vi "GUI Final.vi"() -> ()   [LabVIEW 2014]
uses:
  <vilib>/Instr/_visa.llb/VISA Configure Serial Port (Instr).vi
panel:
  in  "Temperature Threshold":string
  out "read buffer":string
  out "pass ACK":bool
  out "Threshold sent":bool
  out "no of trials read":bool
  out "PC on Ack":bool
  out "Reset#":i32
  in  "Reset":bool
  out "return count read":u32
  in  "VISA resource name":refnum<visa-resource-name>
  out "Iteration":i32
  out "password is wrong":bool
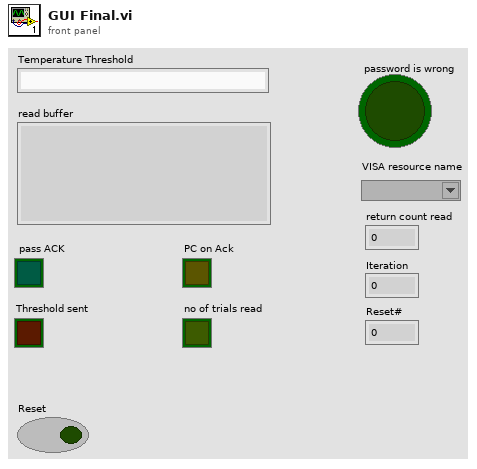
[diagram p1: front panel]
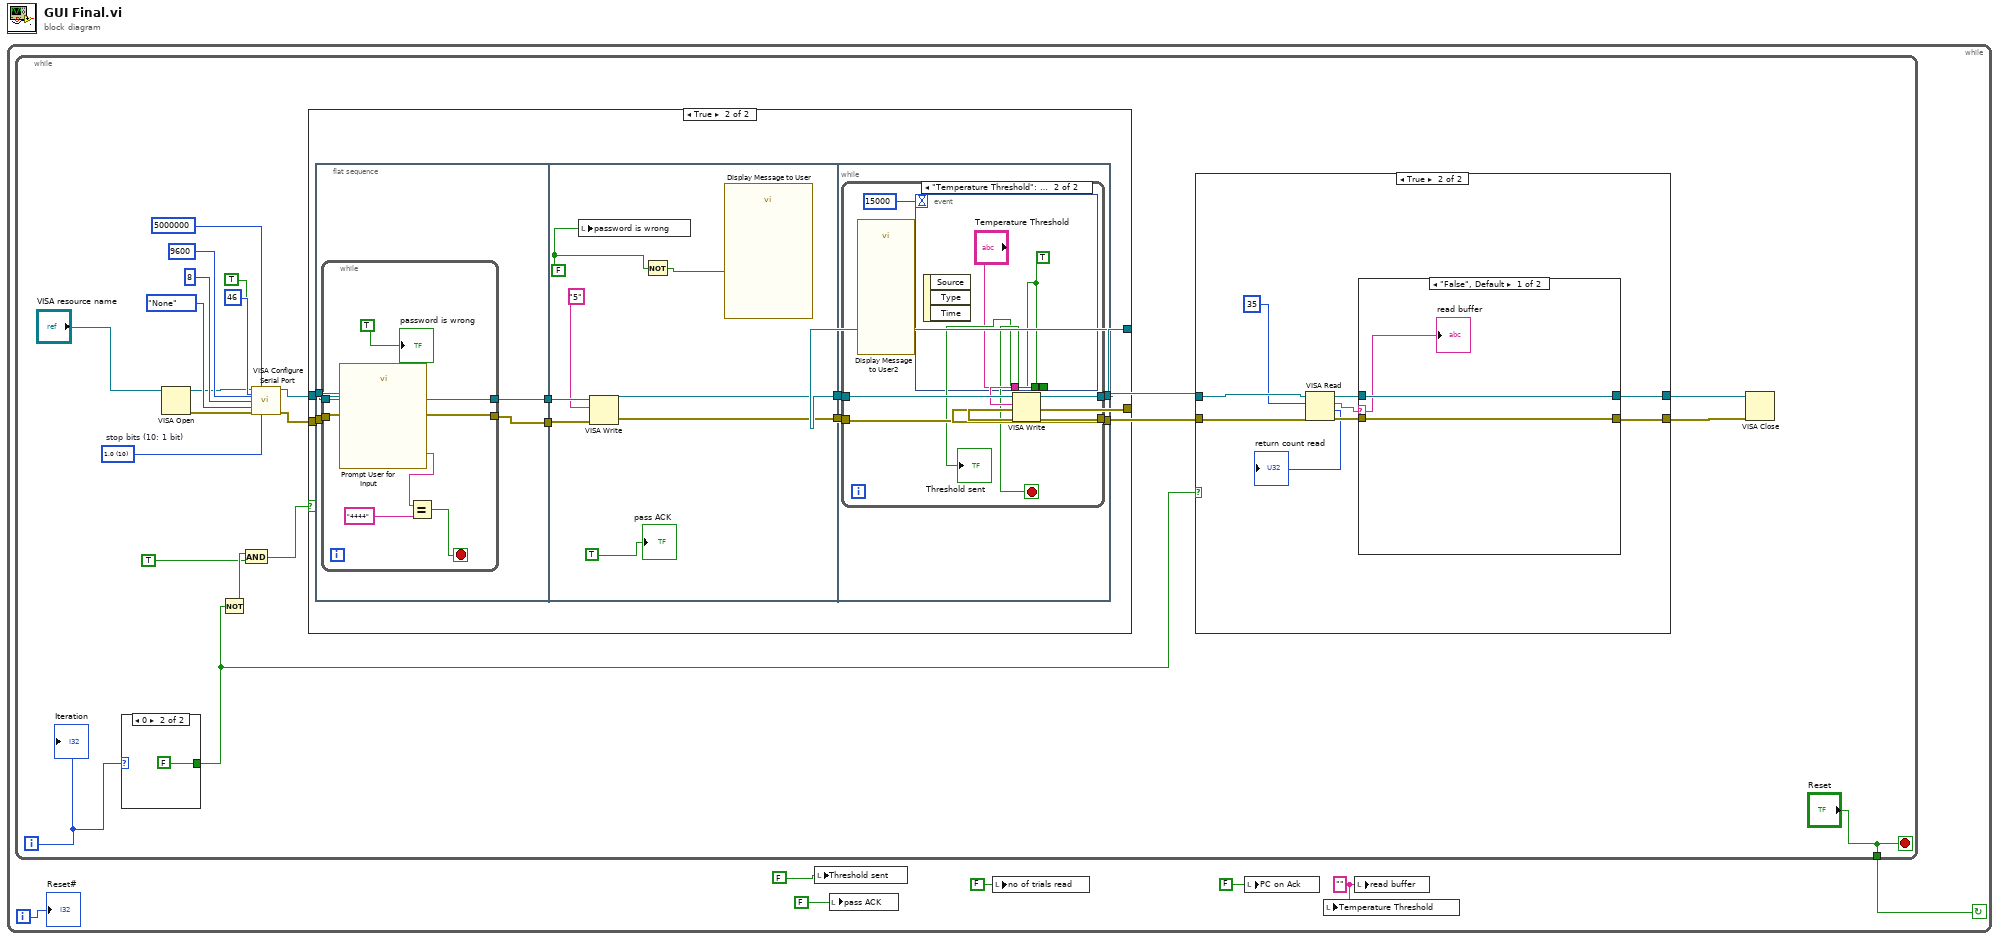
[diagram p0: block diagram]
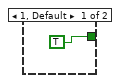
[diagram p2: hidden frame]
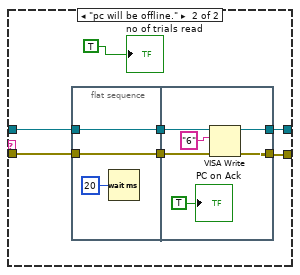
[diagram p4: hidden frame]
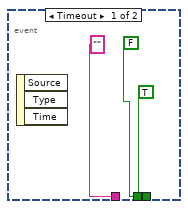
[diagram p6: hidden frame]
diagram:
  n1 = while {
    i -> [w7]
    stop <- w6 continue-if-true
    w1 = "" ("read buffer")
    n2 = while {
      tunnel: ["Reset"] -> w6
      i -> [w15]
      stop <- "Reset" stop-if-true
      w26 = u16 10 items=["1.0"=10, "1.5"=15, "2.0"=20]  # stop bits (10: 1 bit)
      n3 = case shown="0" w15 {
        tunnel: [TRUE FALSE] -> w14
        frame 1, Default {
        }
        frame 0 {
        }
      }
      n4 = VISA Open(VISA resource name="VISA resource name") -> (VISA resource name=w10:refnum<visa-resource-name>, error out=w9:errorcluster)  [unwired: 4 in]
      n5 = Not(x=w14) -> (.not. x?=w23:bool)
      n6 = And(x=w23, y=TRUE) -> (x .and. y?=w20:bool)
      n7 = call-poly "VISA Configure Serial Port"("VISA resource name"=w10, "timeout (10sec)"=u32 5000000, "termination char\n(0xA = '\\n' = LF)"=u8 46 ("termination char\n(0xA = '\\n' = LF)"), "Enable Termination\nChar (T)"=TRUE ("Enable Termination\nChar (T)"), "baud rate (9600)"=u32 9600, "data bits (8)"=u16 8, "parity (0:none)"=enum16{"None", "Odd", "Even", "Mark", "Space"}."None", "error in (no error)"=w9, "stop bits (10: 1 bit)"=w26) -> ("VISA resource name out"=w22:refnum<visa-resource-name>, "error out"=w21:errorcluster)  [unwired: 5 in]
      n8 = case shown="True" w20 {
        tunnel: w21 -> [w63 w71]
        tunnel: [w62 w69] -> w19
        tunnel: [w63 w68] -> w17
        tunnel: w22 -> [w62 w70]
        frame False {
        }
        frame True {
          n9 = flat-sequence {
            tunnel: w71 -> [w75]
            tunnel: w70 -> [w74]
            tunnel: [w73] -> w65
            tunnel: [w72] -> w64
            tunnel: w65 -> [w89]
            tunnel: w64 -> [w88]
            tunnel: [w87] -> w67
            tunnel: [w86] -> w66
            tunnel: [w92] -> w69
            tunnel: [w91] -> w68
            tunnel: w67 -> [w93]
            tunnel: w66 -> [w90]
            frame #0 {
              n10 = while {
                tunnel: w75 -> [w80]
                tunnel: w74 -> [w79]
                tunnel: [w80] -> w73
                tunnel: [w79] -> w72
                stop <- w81 stop-if-true
                n11 = call "Prompt User for Input"() -> ("password"=w76:string)  [unwired: 17 in, 2 out]
                n12 = Equal?(x=w76, y="4444") -> (x = y?=w81:bool)
                "password is wrong" <- TRUE
              }
            }
            frame #1 {
              w83 = FALSE
              n13 = local write "password is wrong"(w83) -> ()
              n14 = VISA Write(VISA resource name=w88, write buffer="5", error in (no error)=w89) -> (VISA resource name out=w87:refnum<visa-resource-name>, error out=w86:errorcluster)  [unwired: 1 out]
              n15 = Not(x=w83) -> (.not. x?=w82:bool)
              n16 = call "Display Message to User"("Enable"=w82) -> ()  [unwired: 9 in, 2 out]
              "pass ACK" <- TRUE ("Pass Ack")
            }
            frame #2 {
              n17 = while {
                tunnel: w93 -> [w101]
                tunnel: [w100] -> w92
                tunnel: [w99] -> w91
                tunnel: w90 -> [w98]
                stop <- w95 stop-if-true
                n18 = call "Display Message to User2"() -> ()  [unwired: 10 in, 2 out]
                n19 = event shown="[1] \"Temperature Threshold\": Value Change" {
                  selector: _ -> [_ _]
                  dyn-events: _ -> [_ _]
                  timeout: 15000 -> [_ _]
                  tunnel: [TRUE w105] -> w95
                  tunnel: ["" "Temperature Threshold"] -> w97
                  tunnel: [FALSE w105] -> w94
                  event Timeout {
                    n20 = event-data() -> ()  [unwired: 1 in, 3 out]
                  }
                  event "Temperature Threshold": Value Change {
                    w105 = TRUE
                    n21 = event-data() -> ()  [unwired: 1 in, 3 out]
                  }
                }
                "Threshold sent" <- w94
                n22 = VISA Write(VISA resource name=w101, write buffer=w97, error in (no error)=w98) -> (VISA resource name out=w100:refnum<visa-resource-name>, error out=w99:errorcluster)  [unwired: 1 out]
              }
            }
          }
        }
      }
      n23 = case shown="True" w14 {
        tunnel: [w33 w41] -> w18
        tunnel: [w32 w42] -> w16
        tunnel: w19 -> [w33 w36]
        tunnel: w17 -> [w32 w35]
        frame False {
        }
        frame True {
          n24 = VISA Read(VISA resource name=w36, byte count=u32 35, error in (no error)=w35) -> (VISA resource name out=w39:refnum<visa-resource-name>, read buffer=w37:string, return count=→"return count read":u32, error out=w40:errorcluster)
          n25 = case shown="\"False\", Default" w37 {
            selector: w37 -> [w43 _]
            tunnel: [w44 w49] -> w42
            tunnel: [w45 w50] -> w41
            tunnel: w40 -> [w44 w51]
            tunnel: w39 -> [w45 w52]
            frame "False", Default {
              "read buffer" <- w43
            }
            frame "pc will be offline." {
              n26 = flat-sequence {
                tunnel: w51 -> [w54]
                tunnel: w52 -> [w55]
                tunnel: [w55] -> w48
                tunnel: [w54] -> w47
                tunnel: [w59] -> w50
                tunnel: [w58] -> w49
                tunnel: w48 -> [w61]
                tunnel: w47 -> [w60]
                frame #0 {
                  n27 = Wait (ms)(milliseconds to wait=u32 20) -> ()  [unwired: 1 out]
                }
                frame #1 {
                  n28 = VISA Write(VISA resource name=w61, write buffer="6", error in (no error)=w60) -> (VISA resource name out=w59:refnum<visa-resource-name>, error out=w58:errorcluster)  [unwired: 1 out]
                  "PC on Ack" <- TRUE ("PC on Ack")
                }
              }
              "no of trials read" <- TRUE ("PC on Ack")
            }
          }
        }
      }
      n29 = VISA Close(VISA resource name=w18, error in (no error)=w16) -> ()  [unwired: 1 out]
      "Iteration" <- w15
    }
    n30 = local write "Threshold sent"(FALSE) -> ()
    n31 = local write "pass ACK"(FALSE ("Pass Ack")) -> ()
    n32 = local write "no of trials read"(FALSE ("no of trials read")) -> ()
    n33 = local write "PC on Ack"(FALSE) -> ()
    n34 = local write "Temperature Threshold"(w1) -> ()
    n35 = local write "read buffer"(w1) -> ()
    "Reset#" <- w7
  }
